vi "NewGame.vi"(7 "SnakeGameType (ChildObject)":refnum<class "SnakeGame.lvclass">, 8 "error in (no error)":errorcluster, 11 "FPGA_ref":T1) -> (0 "error out":errorcluster, 3 "SnakeGame out":refnum<class "SnakeGame.lvclass">)   [LabVIEW 2019, in "RT_Game.lvlib" / "SnakeGame.lvclass"]
uses:
  SnakeGame.lvclass
  C:/Users/FreshBob/Dropbox/VIs/myRIO_GameConsole/RT/RT_Game/Game/Game.lvclass
  FPGA_Interface.ctl
  RT_Sprite/RT_Sprite.lvclass
  C:/Users/FreshBob/Dropbox/VIs/myRIO_GameConsole/RT/RT_Game/GameObject/GameObject.lvclass
  Game/Coordinate.ctl
  PongSwitch/SnakeSwitch.lvclass
  Snake/Direction.ctl
  Snake/Snake.lvclass
  Snake/Snake.lvclass/Snake.ctl
  GameObject/GameObject.lvclass/GameObject.ctl
  PongSwitch/SnakeSwitch.lvclass/SnakeSwitch.ctl
  Game/Game.lvclass/Game.ctl
  SnakeGame.lvclass/SnakeGame.ctl
  GameObject/Write name.vi
  PongSwitch/Write Static.vi
  GameObject/Write IsActive.vi
  PongSwitch/Write Tilecode.vi
  GameObject/Read position.vi
  Snake/Write Position (Tiles).vi
  Snake/Write Direction.vi
  Snake/Write ScorePosition.vi
  Snake/Write Color.vi
  Snake/Write Length.vi
  Snake/Write tick_rate.vi
  PongSwitch/Write DisabledTime.vi
  PongSwitch/Write EnabledTime.vi
  PongSwitch/Write randomness.vi
  GameObject/Write Collides_.vi
  Game/Read Singleplayer.vi
  Snake/Write Dead_.vi
  Game/Write Sprites.vi
  Game/Game.lvclass
  GameObject/GameObject.lvclass
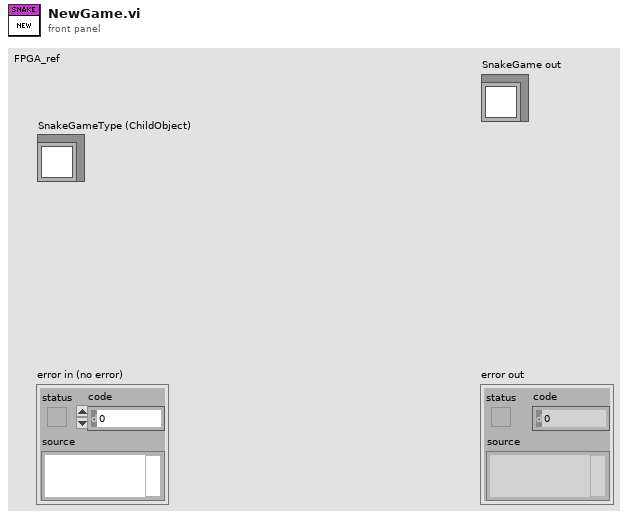
[diagram p1: front panel]
types:
  T1 = typedef "FPGA_Interface.ctl" = refnum<k20>
  T2 = typedef "RT_Game.lvlib/Game.lvclass/Coordinate.ctl" = cluster{"x":dbl, "y":dbl}
  T3 = typedef "RT_Game.lvlib/Snake.lvclass/Direction.ctl" = enum16{"Up", "Left", "Down", "Right"}
  T4 = cluster{"GameObject out":refnum<class "RT_Sprite.lvclass">, "GameObject out":refnum<class "RT_Sprite.lvclass">, "GameObject out":refnum<class "RT_Sprite.lvclass">}
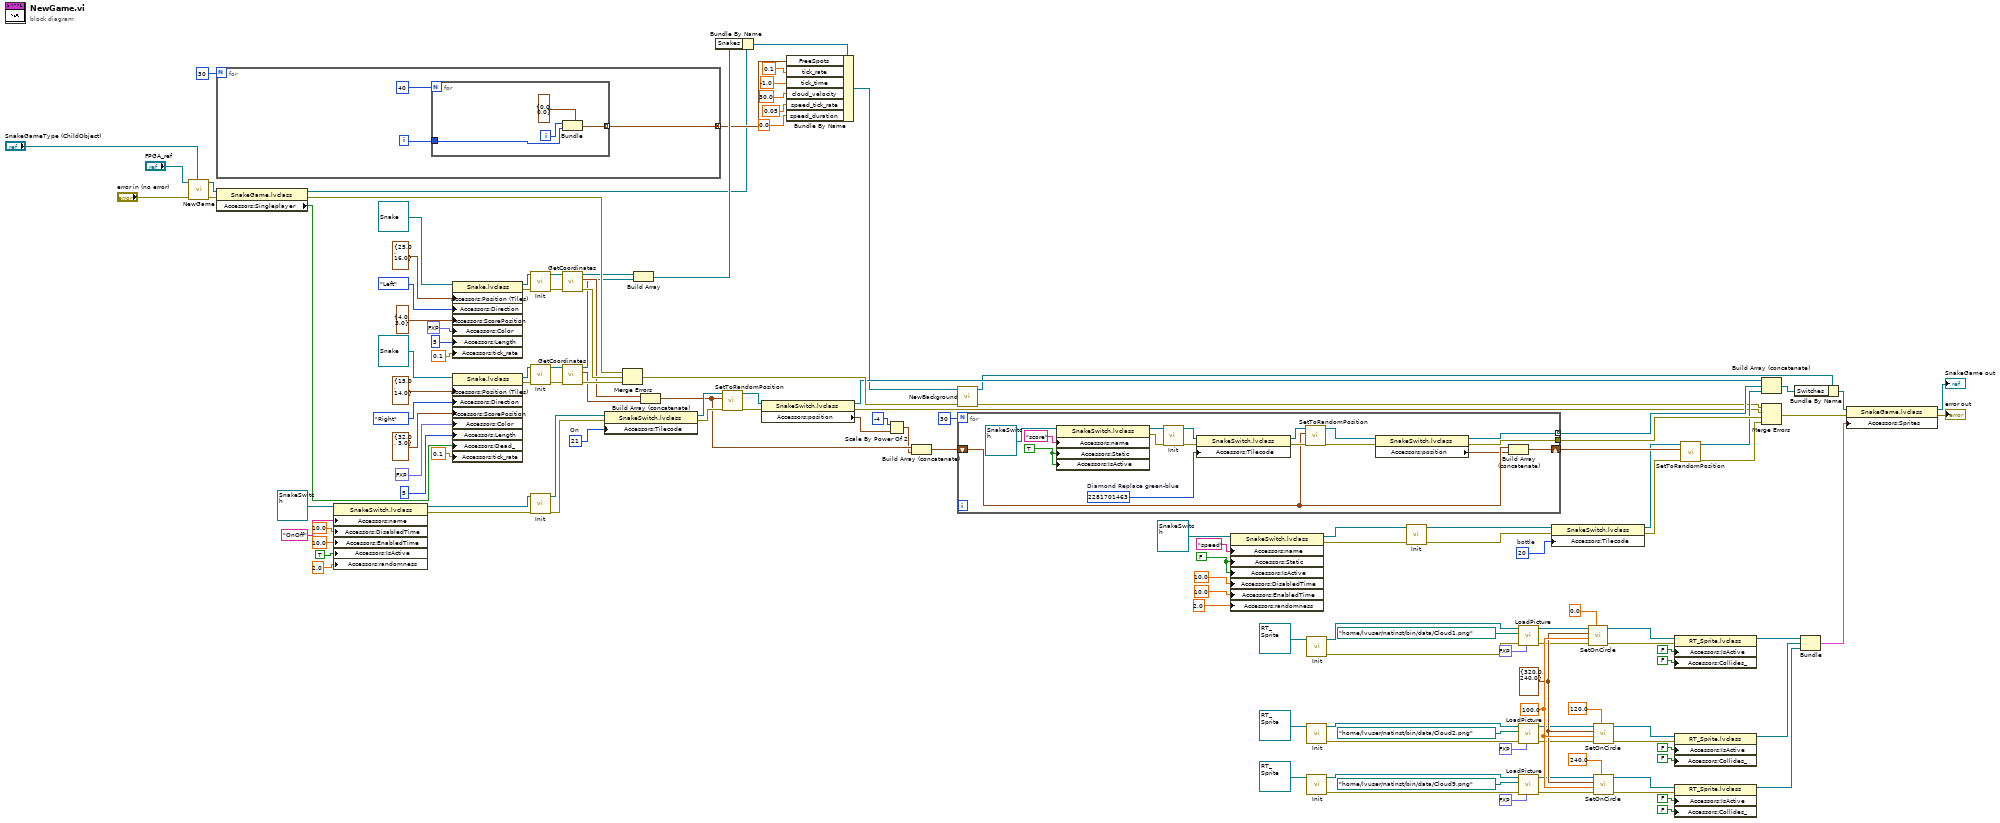
[diagram p0: block diagram]
diagram:
  w130 = u32 21  # On
  w126 = u32 20  # bottle
  w72 = FALSE ("Static")
  w64 = 100.0 ("Radius")
  w63 = T2 {"x"=320.0, "y"=240.0} ("Center")
  n1 = call-parent "NewGame.vi"("GameType (ChildObject)"="SnakeGameType (ChildObject)", "error in (no error)"="error in (no error)", "FPGA_ref"="FPGA_ref") -> ("error out"=w4:errorcluster, "Game out"=w5:refnum<class "SnakeGame.lvclass">)  [unwired: 7 in]
  n2 = for {
    N: 30 -> [_]
    tunnel: [w138] -> w88 mode=concatenating
    i -> [w139]
    n3 = for {
      N: 40 -> [_]
      tunnel: w139 -> [w142]
      tunnel: [w141] -> w138 mode=indexing
      i -> [w143]
      n4 = Bundle(cluster=T2 {"x"=0.0, "y"=0.0} ("Coordinate"), "x"=w143, "y"=w142) -> (w141:T2)
    }
  }
  n5 = property class="SnakeGame.lvclass"(reference=w5, error in=w4) -> (reference out=w1:refnum<class "SnakeGame.lvclass">, error out=w133:errorcluster, "Accessors:Singleplayer"=w134:bool)
  n6 = property class="SnakeSwitch.lvclass"(reference=refnum<class "SnakeSwitch.lvclass"> refnum ("RT_Game.lvlib:SnakeSwitch.lvclass"), "Accessors:name"="OnOff" ("name"), "Accessors:DisabledTime"=10.0 ("DisabledTime"), "Accessors:EnabledTime"=10.0 ("EnabledTime"), "Accessors:IsActive"=TRUE ("IsActive"), "Accessors:randomness"=2.0 ("randomness")) -> (reference out=w19:refnum<class "SnakeSwitch.lvclass">, error out=w21:errorcluster)  [unwired: 1 in]
  n7 = property class="Snake.lvclass"(reference=refnum<class "Snake.lvclass"> refnum ("RT_Game.lvlib:Snake.lvclass"), "Accessors:Position (Tiles)"=T2 {"x"=25.0, "y"=16.0} ("Position (Tiles)"), "Accessors:Direction"=Direction."Left" ("Direction"), "Accessors:ScorePosition"=T2 {"x"=4.0, "y"=3.0} ("ScorePosition"), "Accessors:Color"=fxp<+,3,3> 1.0 ("Color"), "Accessors:Length"=i16 5 ("Length"), "Accessors:tick_rate"=0.1 ("tick_rate")) -> (reference out=w92:refnum<class "Snake.lvclass">, error out=w93:errorcluster)  [unwired: 1 in]
  n8 = property class="Snake.lvclass"(reference=refnum<class "Snake.lvclass"> refnum ("RT_Game.lvlib:Snake.lvclass"), "Accessors:Position (Tiles)"=T2 {"x"=15.0, "y"=14.0} ("Position (Tiles)"), "Accessors:Direction"=Direction."Right" ("Direction"), "Accessors:ScorePosition"=T2 {"x"=32.0, "y"=3.0} ("ScorePosition"), "Accessors:Color"=fxp<+,3,3> 2.0 ("Color"), "Accessors:Length"=i16 5 ("Length"), "Accessors:Dead_"=w134, "Accessors:tick_rate"=0.1 ("tick_rate")) -> (reference out=w105:refnum<class "Snake.lvclass">, error out=w104:errorcluster)  [unwired: 1 in]
  n9 = call-dynamic "Init.vi"("error in (no error)"=w93, "Snake in"=w92) -> ("error out"=w119:errorcluster, "Snake out"=w108:refnum<class "Snake.lvclass">)  [unwired: 8 in]
  n10 = call-dynamic "Init.vi"("error in (no error)"=w104, "Snake in"=w105) -> ("error out"=w121:errorcluster, "Snake out"=w109:refnum<class "Snake.lvclass">)  [unwired: 8 in]
  n11 = call-dynamic "Init.vi"("error in (no error)"=w21, "PongSwitch in"=w19) -> ("error out"=w17:errorcluster, "PongSwitch out"=w128:refnum<class "SnakeSwitch.lvclass">)  [unwired: 8 in]
  n12 = call "GetCoordinates.vi"("error in (no error)"=w119, "Snake in"=w108) -> ("error out"=w120:errorcluster, "Coordinates"=w116:T2[], "Snake out"=w114:refnum<class "Snake.lvclass">)  [unwired: 7 in]
  n13 = call "GetCoordinates.vi"("error in (no error)"=w121, "Snake in"=w109) -> ("error out"=w122:errorcluster, "Coordinates"=w117:T2[], "Snake out"=w115:refnum<class "Snake.lvclass">)  [unwired: 7 in]
  n14 = property class="SnakeSwitch.lvclass"(reference=w128, error in=w17, "Accessors:Tilecode"=w130) -> (reference out=w129:refnum<class "SnakeSwitch.lvclass">, error out=w127:errorcluster)
  n15 = Merge Errors(w133, w120, w122) -> (w110:errorcluster)
  n16 = Build Array(w114, w115) -> (w111:refnum<class "Snake.lvclass">[])
  n17 = Build Array (concatenate)(w116, w117) -> (w118:T2[])
  n18 = Bundle By Name(cluster=w1, "Snakes"=w111) -> (w107:refnum<class "SnakeGame.lvclass">)
  n19 = call "SetToRandomPosition.vi"("error in (no error)"=w127, "BlockedSpots"=w118, "SnakeSwitch in"=w129) -> ("error out"=w22:errorcluster, "SnakeSwitch out"=w28:refnum<class "SnakeSwitch.lvclass">)  [unwired: 7 in]
  n20 = property class="SnakeSwitch.lvclass"(reference=w28, error in=w22) -> (reference out=w29:refnum<class "SnakeSwitch.lvclass">, error out=w27:errorcluster, "Accessors:position"=w30:T2)
  n21 = Bundle By Name(cluster=w107, "FreeSpots"=w88, "tick_rate"=0.1, "tick_time"=-1.0, "cloud_velocity"=30.0, "speed_tick_rate"=0.05, "speed_duration"=0.0) -> (w6:refnum<class "SnakeGame.lvclass">)
  n22 = Scale By Power Of 2(n=i16 -4, x=w30) -> (x*2^n=w32:T2)
  n23 = Build Array (concatenate)(w118, w32) -> (w82:T2[])
  n24 = call "NewBackground.vi"("error in (no error)"=w110, "Snake in"=w6) -> ("error out"=w24:errorcluster, "Snake out"=w26:refnum<class "SnakeGame.lvclass">)  [unwired: 8 in]
  n25 = for {
    N: 30 -> [_]
    tunnel: [w155] -> w80
    tunnel: [w153] -> w81 mode=indexing
    shift-right: [w146] -> w131
    shift-left: w82 -> [w147]
    w148 = u32 2281701463  # Diamond Replace green-blue
    w152 = TRUE ("Static")
    n26 = property class="SnakeSwitch.lvclass"(reference=refnum<class "SnakeSwitch.lvclass"> refnum ("RT_Game.lvlib:SnakeSwitch.lvclass"), "Accessors:name"="score" ("name"), "Accessors:Static"=w152, "Accessors:IsActive"=w152) -> (reference out=w159:refnum<class "SnakeSwitch.lvclass">, error out=w157:errorcluster)  [unwired: 1 in]
    n27 = call-dynamic "Init.vi"("error in (no error)"=w157, "PongSwitch in"=w159) -> ("error out"=w161:errorcluster, "PongSwitch out"=w150:refnum<class "SnakeSwitch.lvclass">)  [unwired: 8 in]
    n28 = property class="SnakeSwitch.lvclass"(reference=w150, error in=w161, "Accessors:Tilecode"=w148) -> (reference out=w149:refnum<class "SnakeSwitch.lvclass">, error out=w151:errorcluster)
    n29 = call "SetToRandomPosition.vi"("error in (no error)"=w151, "BlockedSpots"=w147, "SnakeSwitch in"=w149) -> ("error out"=w156:errorcluster, "SnakeSwitch out"=w154:refnum<class "SnakeSwitch.lvclass">)  [unwired: 7 in]
    n30 = property class="SnakeSwitch.lvclass"(reference=w154, error in=w156) -> (reference out=w153:refnum<class "SnakeSwitch.lvclass">, error out=w155:errorcluster, "Accessors:position"=w145:T2)
    n31 = Build Array (concatenate)(w147, w145) -> (w146:T2[])
  }
  n32 = property class="SnakeSwitch.lvclass"(reference=refnum<class "SnakeSwitch.lvclass"> refnum ("RT_Game.lvlib:SnakeSwitch.lvclass"), "Accessors:name"="speed" ("name"), "Accessors:Static"=w72, "Accessors:IsActive"=w72, "Accessors:DisabledTime"=10.0 ("DisabledTime"), "Accessors:EnabledTime"=10.0 ("EnabledTime"), "Accessors:randomness"=2.0 ("randomness")) -> (reference out=w75:refnum<class "SnakeSwitch.lvclass">, error out=w73:errorcluster)  [unwired: 1 in]
  n33 = call-dynamic "Init.vi"("RT_Sprite in"=refnum<class "RT_Sprite.lvclass"> refnum ("RT_Game.lvlib:RT_Sprite.lvclass")) -> ("error out"=w10:errorcluster, "RT_Sprite out"=w9:refnum<class "RT_Sprite.lvclass">)  [unwired: 9 in]
  n34 = call-dynamic "Init.vi"("RT_Sprite in"=refnum<class "RT_Sprite.lvclass"> refnum ("RT_Game.lvlib:RT_Sprite.lvclass")) -> ("error out"=w36:errorcluster, "RT_Sprite out"=w37:refnum<class "RT_Sprite.lvclass">)  [unwired: 9 in]
  n35 = call-dynamic "Init.vi"("RT_Sprite in"=refnum<class "RT_Sprite.lvclass"> refnum ("RT_Game.lvlib:RT_Sprite.lvclass")) -> ("error out"=w41:errorcluster, "RT_Sprite out"=w40:refnum<class "RT_Sprite.lvclass">)  [unwired: 9 in]
  n36 = call-dynamic "Init.vi"("error in (no error)"=w73, "PongSwitch in"=w75) -> ("error out"=w77:errorcluster, "PongSwitch out"=w124:refnum<class "SnakeSwitch.lvclass">)  [unwired: 8 in]
  n37 = call "LoadPicture.vi"("Transparent Color"=fxp<+,3,3> 0.0, "error in (no error)"=w10, "Picture Path"=path "/home/lvuser/natinst/bin/data/Cloud1.png" ("Tile Path"), "RT_Sprite in"=w9) -> ("error out"=w13:errorcluster, "RT_Sprite out"=w47:refnum<class "RT_Sprite.lvclass">)  [unwired: 6 in]
  n38 = call "LoadPicture.vi"("Transparent Color"=fxp<+,3,3> 0.0, "error in (no error)"=w36, "Picture Path"=path "/home/lvuser/natinst/bin/data/Cloud2.png" ("Tile Path"), "RT_Sprite in"=w37) -> ("error out"=w48:errorcluster, "RT_Sprite out"=w34:refnum<class "RT_Sprite.lvclass">)  [unwired: 6 in]
  n39 = call "LoadPicture.vi"("Transparent Color"=fxp<+,3,3> 0.0, "error in (no error)"=w41, "Picture Path"=path "/home/lvuser/natinst/bin/data/Cloud9.png" ("Tile Path"), "RT_Sprite in"=w40) -> ("error out"=w43:errorcluster, "RT_Sprite out"=w61:refnum<class "RT_Sprite.lvclass">)  [unwired: 6 in]
  n40 = property class="SnakeSwitch.lvclass"(reference=w124, error in=w77, "Accessors:Tilecode"=w126) -> (reference out=w125:refnum<class "SnakeSwitch.lvclass">, error out=w123:errorcluster)
  n41 = call "SetOnCircle.vi"("angle (deg)"=0.0, "error in (no error)"=w13, "Radius"=w64, "Center"=w63, "GameObject in"=w47) -> ("error out"=w57:errorcluster, "GameObject out"=w56:refnum<class "RT_Sprite.lvclass">)  [unwired: 5 in]
  n42 = call "SetOnCircle.vi"("angle (deg)"=120.0, "error in (no error)"=w48, "Radius"=w64, "Center"=w63, "GameObject in"=w34) -> ("error out"=w59:errorcluster, "GameObject out"=w58:refnum<class "RT_Sprite.lvclass">)  [unwired: 5 in]
  n43 = call "SetOnCircle.vi"("angle (deg)"=240.0, "error in (no error)"=w43, "Radius"=w64, "Center"=w63, "GameObject in"=w61) -> ("error out"=w60:errorcluster, "GameObject out"=w62:refnum<class "RT_Sprite.lvclass">)  [unwired: 5 in]
  n44 = property class="RT_Sprite.lvclass"(reference=w56, error in=w57, "Accessors:IsActive"=FALSE ("IsActive"), "Accessors:Collides_"=FALSE ("Collides_")) -> (reference out=w53:refnum<class "RT_Sprite.lvclass">)  [unwired: 1 out]
  n45 = property class="RT_Sprite.lvclass"(reference=w58, error in=w59, "Accessors:IsActive"=FALSE ("IsActive"), "Accessors:Collides_"=FALSE ("Collides_")) -> (reference out=w54:refnum<class "RT_Sprite.lvclass">)  [unwired: 1 out]
  n46 = property class="RT_Sprite.lvclass"(reference=w62, error in=w60, "Accessors:IsActive"=FALSE ("IsActive"), "Accessors:Collides_"=FALSE ("Collides_")) -> (reference out=w55:refnum<class "RT_Sprite.lvclass">)  [unwired: 1 out]
  n47 = call "SetToRandomPosition.vi"("error in (no error)"=w123, "BlockedSpots"=w131, "SnakeSwitch in"=w125) -> ("error out"=w78:errorcluster, "SnakeSwitch out"=w79:refnum<class "SnakeSwitch.lvclass">)  [unwired: 7 in]
  n48 = Build Array (concatenate)(w29, w81, w79) -> (w18:refnum<class "SnakeSwitch.lvclass">[])
  n49 = Merge Errors(w24, w27, w80, w78) -> (w25:errorcluster)
  n50 = Bundle By Name(cluster=w26, "Switches"=w18) -> (w23:refnum<class "SnakeGame.lvclass">)
  n51 = Bundle("GameObject out"=w53, "GameObject out"=w54, "GameObject out"=w55) -> (w12:T4)  [unwired: 1 in]
  n52 = property class="SnakeGame.lvclass"(reference=w23, error in=w25, "Accessors:Sprites"=w12) -> (reference out=→"SnakeGame out":refnum<class "SnakeGame.lvclass">, error out=→"error out":errorcluster)
